vi "ROI group-Auto scroll.vi"(8 "error in (no error)":errorcluster, 9 "Array":T2[](array[typedef]), 11 "[Groups]":T1) -> (0 "error out":errorcluster)   [LabVIEW 2020]
uses:
  Typedefs/Group sel cluster.ctl
  Typedefs/Groups array referecne.ctl
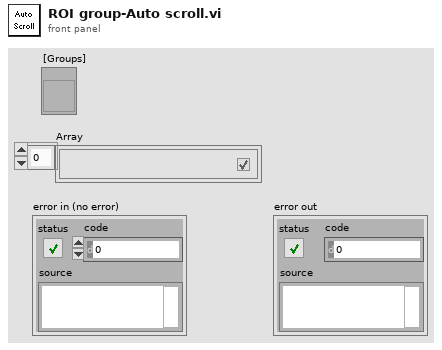
[diagram p1: front panel]
types:
  T1 = typedef "Groups array referecne.ctl" = refnum<vi>
  T2 = typedef "Group sel cluster.ctl" = cluster{"Group number":string, "Group Name":string, "Visibility":bool, "Highlight":bool}
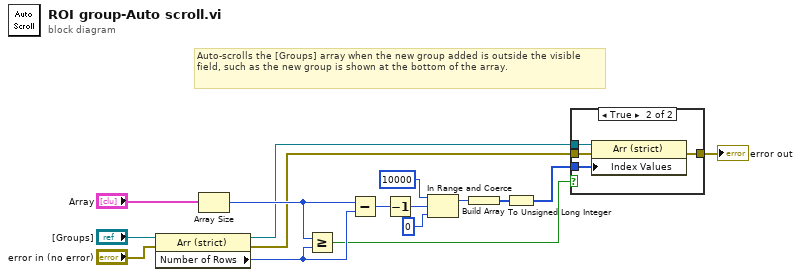
[diagram p0: block diagram]
diagram:
  # "Auto-scrolls the [Groups] array when the new group added is outside the visible field, such as the new group is shown at the bottom of the array."
  n1 = property on="Property Node" class="Arr (strict)"(reference="[Groups]", error in="error in (no error)") -> (reference out=w4:T1, error out=w2:errorcluster, "Number of Rows"=w16:u32)
  n2 = Array Size(array="Array") -> (size(s)=w14:i32)
  n3 = Greater Or Equal?(x=w14, y=w16) -> (x >= y?=w13:bool)
  n4 = Subtract(x=w14, y=w16) -> (x-y=w15:u32)
  n5 = Decrement(x=w15) -> (x-1=w5:u32)
  n6 = In Range and Coerce(upper limit=10000, x=w5, lower limit=0) -> (coerced(x)=w8:u32)  [unwired: 1 out]
  n7 = Build Array(w8) -> (w9:u32[])
  n8 = To Unsigned Long Integer(number=w9) -> (unsigned 32bit integer=w12:u32[])
  n9 = case shown="True" w13 {
    tunnel: w2 -> [w17 w21]
    tunnel: [w17 w20] -> w11
    tunnel: w12 -> [_ w19]
    tunnel: w4 -> [_ w18]
    frame False {
    }
    frame True {
      n10 = property on="Property Node" class="Arr (strict)"(reference=w18, error in=w21, "Index Values"=w19) -> (error out=w20:errorcluster)  [unwired: 1 out]
    }
  }
  "error out" <- w11
